vi "FormatRanges.vi"(11 "cluster":T1) -> (3 "range string array":string[][](array[string]))   [LabVIEW 2016]
doc: "VI that formats the saved ranges (weak left through strong right) to add to the end of the data file."
uses:
  DataLoopCluster.ctl
  SignalType.ctl
  range_cluster.ctl
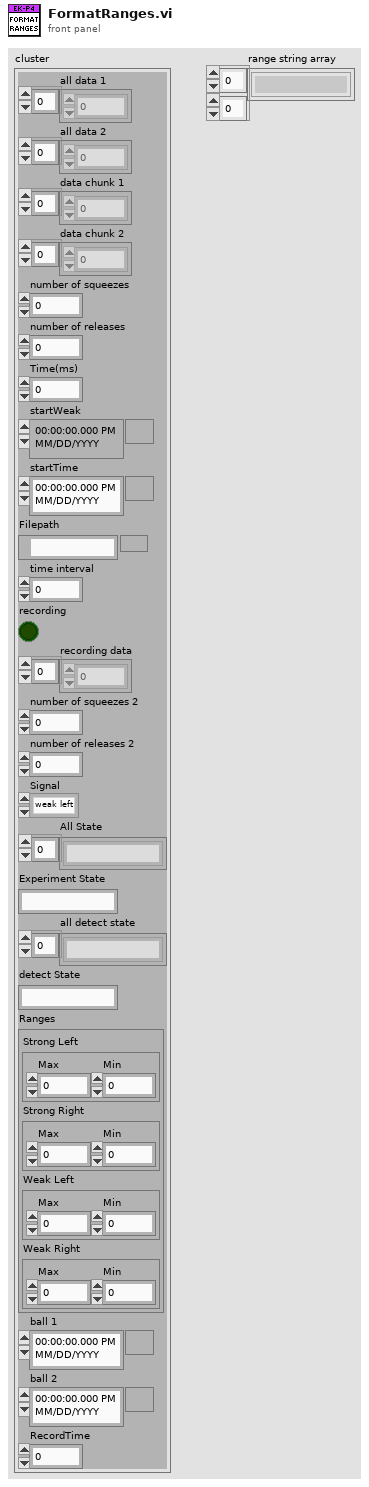
[diagram p1: front panel]
types:
  T1 = typedef "DataLoopCluster.ctl" = cluster{"all data 1":dbl[], "all data 2":dbl[], "data chunk 1":dbl[], "data chunk 2":dbl[], "number of squeezes":u16, "number of releases":u16, "Time(ms)":i64, "startWeak":timestamp, "startTime":timestamp, "Filepath":path, "time interval":u16, "recording":bool, "recording data":dbl[], "number of squeezes 2":u16, "number of releases 2":u16, "Signal":T2, "All State":string[], "Experiment State":string, "all detect state":string[], "detect State":string, "Ranges":cluster{"Strong Left":T3, "Strong Right":T3, "Weak Left":T3, "Weak Right":T3}, "ball 1":timestamp, "ball 2":timestamp, "RecordTime":u16}
  T2 = typedef "SignalType.ctl" = enum16{"weak left", "weak right", "strong left", "strong right"}
  T3 = typedef "range_cluster.ctl" = cluster{"Max":dbl, "Min":dbl}
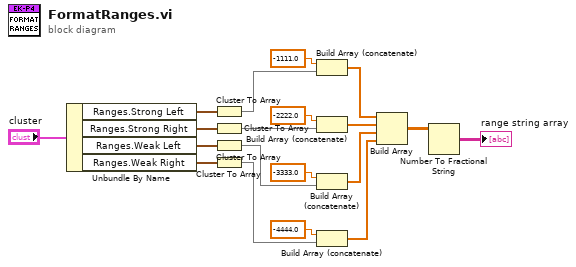
[diagram p0: block diagram]
diagram:
  n1 = Unbundle By Name("cluster") -> ("Ranges.Strong Left"=w12:T3, "Ranges.Strong Right"=w10:T3, "Ranges.Weak Left"=w6:T3, "Ranges.Weak Right"=w3:T3)
  n2 = Cluster To Array(cluster=w12) -> (array=w11:dbl[])
  n3 = Cluster To Array(cluster=w10) -> (array=w9:dbl[])
  n4 = Cluster To Array(cluster=w6) -> (array=w8:dbl[])
  n5 = Cluster To Array(cluster=w3) -> (array=w2:dbl[])
  n6 = Build Array (concatenate)(-1111.0 ("element"), w11) -> (w14:dbl[])
  n7 = Build Array (concatenate)(-2222.0 ("element"), w9) -> (w15:dbl[])
  n8 = Build Array (concatenate)(-3333.0 ("element"), w8) -> (w5:dbl[])
  n9 = Build Array (concatenate)(-4444.0 ("element"), w2) -> (w1:dbl[])
  n10 = Build Array(w14, w15, w5, w1) -> (w17:dbl[][])
  n11 = Number To Fractional String(number=w17) -> (F-format string=→"range string array":string[][])  [unwired: 3 in]
